vi "Close All COM Ports.vi"   [LabVIEW 2014]
uses:
  Aircraft Information/Sub VI/Get Aircraft Information.vi
types:
  T1 = typedef "Drone Information.ctl" = cluster{"Heart Beat":bool, "Aircraft ID":u8, "Downlink Port":refnum<visa-resource-name>, "Tag ID":string, "System Status":string, "Base Mode":T2, "Armed/Disarmed":bool, "Battery Voltage":dbl, "Control Mode":T3, "Initialisation":u8, "Heart Beat Status":bool, "Uplink Port":refnum<visa-resource-name>, "UDP connection ID":refnum<k16>, "Connection Type":T4, "Mode":string, "UDP IP Address":string, "Mission Uploaded":bool}
  T2 = typedef "Base Mode.ctl" = cluster{"Custom Mode":bool, "Test Enabled":bool, "Autonomous Mode":bool, "Guided Mode":bool, "Stabilization Enabled":bool, "HIL Enabled":bool, "Manual Mode":bool, "Arm":bool}
  T3 = typedef "Aircraft Mode.ctl" = enum16{"Loiter", "Stabalise", "Failsafe", "Emergency Stop"}
  T4 = typedef "Telemetry Connection Type.ctl" = enum16{"Serial", "UDP", "TCP"}
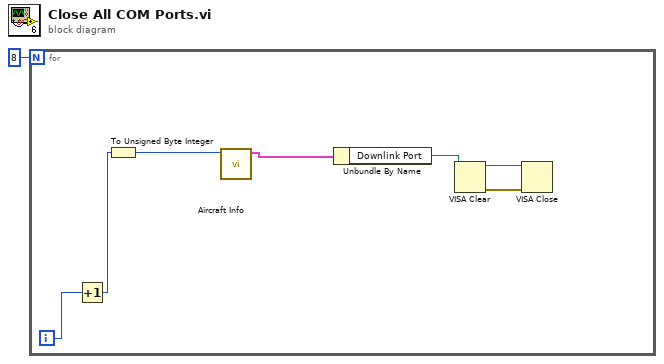
[diagram p0: block diagram]
diagram:
  n1 = for {
    N: 8 -> [_]
    i -> [w8]
    n2 = Increment(x=w8) -> (x+1=w6:i32)
    n3 = To Unsigned Byte Integer(number=w6) -> (unsigned 8bit integer=w7:u8)
    n4 = call-poly "Aircraft Info.vi"("Aircraft ID"=w7) -> ("Aircraft Information Out"=w2:T1)  [unwired: 9 in, 1 out]
    n5 = Unbundle By Name(w2) -> ("Downlink Port"=w3:refnum<visa-resource-name>)
    n6 = VISA Clear(VISA resource name=w3) -> (VISA resource name out=w5:refnum<visa-resource-name>, error out=w4:errorcluster)  [unwired: 1 in]
    n7 = VISA Close(VISA resource name=w5, error in (no error)=w4) -> ()  [unwired: 1 out]
  }
